vi "GetInstance.vi"(8 "Error In":errorcluster {"Code" format="%.0x"}, 11 "Core In":refnum<class "Core.lvclass">) -> (0 "Error Out":errorcluster {"Code" format="%.0x"}, 2 "Instance":refnum<vi>, 3 "Core Out":refnum<class "Core.lvclass">)   [LabVIEW 2020, in "Core.lvlib" / "Core.lvclass"]
doc: "Property for reading <B>Instance</B> from internal data structure for current object instance."
uses:
  Core.lvclass
  DataReference.ctl
  Data.ctl
  Build.ctl
  Core.lvclass/Core.ctl
panel:
  # "/* Inputs */"
  # "/* Locals */"
  # "/* Outputs */"
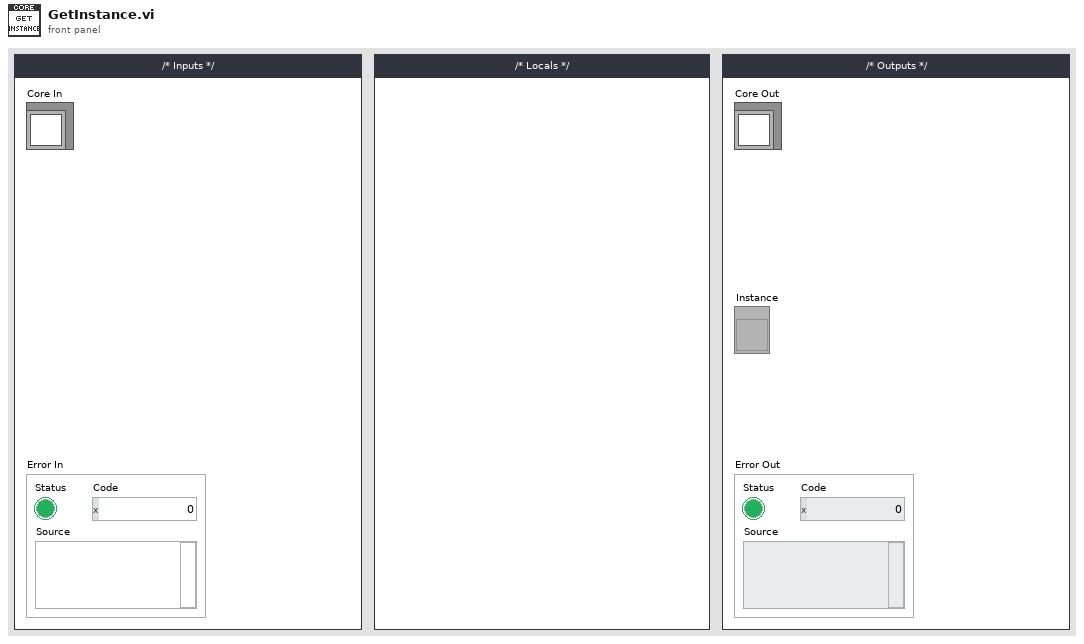
[diagram p1: front panel]
types:
  T1 = typedef "Core.lvlib/Core.lvclass/DataReference.ctl" = refnum<data-value>
  T2 = typedef "Core.lvlib/Core.lvclass/Data.ctl" = cluster{"Core":refnum<class "Core.lvclass">, "Instance":refnum<vi>, "Name":string, "Namespace":string, "Build":T3}
  T3 = typedef "Core.lvlib/Core.lvclass/Build.ctl" = cluster{"Computer":string, "PlatformOS":string, "PlatformVer":string, "Timestamp":string, "Version":string, "Author":string, "Company":string, "GUID":string}
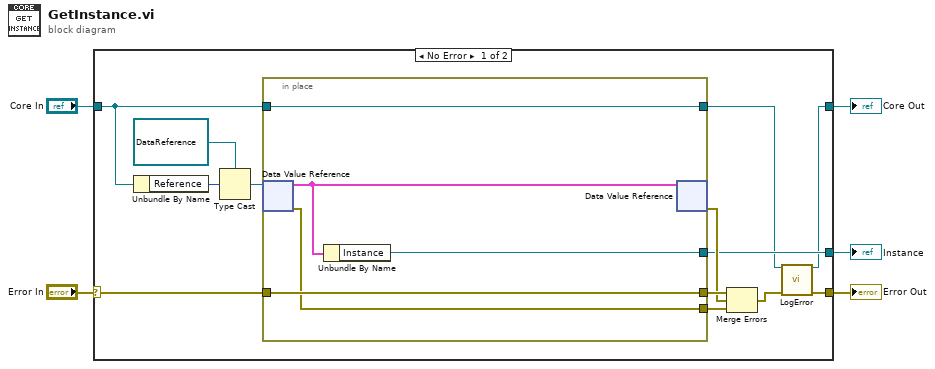
[diagram p0: block diagram]
diagram:
  n1 = case shown="No Error" "Error In" {
    selector: "Error In" -> [w16 w24]
    tunnel: [w8 w24] -> w4
    tunnel: "Core In" -> [w14 w25]
    tunnel: [w7 w25] -> w2
    tunnel: [w10 _] -> w1
    frame No Error {
      n2 = Unbundle By Name(w14) -> ("Reference"=w18:u64)
      n3 = Type Cast(type=T1 refnum ("Data Reference"), x=w18) -> (*(type *) &x=w15:T1)
      n4 = in-place {
        in-place-border: w16 -> [w22]
        in-place-border: w14 -> [w23]
        in-place-border: [w23] -> w6
        in-place-border: [w22] -> w13
        in-place-border: [w21] -> w11
        in-place-border: [w19] -> w10
        n5 = in-place-dvr #1(w15) -> (w20:T2, w21:errorcluster)
        n6 = Unbundle By Name(w20) -> ("Instance"=w19:refnum<vi>)
        n7 = in-place-dvr #1(w20) -> (w12:errorcluster)  [unwired: 1 out]
      }
      n8 = Merge Errors(w13, w12, w11) -> (w9:errorcluster)
      n9 = call-dynamic "LogError.vi"("Core In"=w6, "Error In"=w9) -> ("Core Out"=w7:refnum<class "Core.lvclass">, "Error Out"=w8:errorcluster)  [unwired: 12 in]
    }
    frame Error {
    }
  }
  "Core Out" <- w2
  "Error Out" <- w4
  "Instance" <- w1
